vi "MB ICPCON Param redefine.vi"(6 "conninfo":T3={"host"="localhost", "port"="5432", "client_encoding"="WIN1251", "dbname"="data", "user"="postgres", "password"=""}, 7 "Status Reference":T1, 8 "error in (no error)":errorcluster, 9 "KFMTable":string="kfm_3", 10 "KFM param":string[](array[string]), 11 "KFM param in":T2) -> (0 "error":errorcluster, 3 "KFM param out":T2, 5 "Status Reference out":T1)   [LabVIEW 2019, in "ICPCON_Param.lvlib"]
uses:
  ICPCON_Param.lvlib
  ICPCON Param.ctl
  Eth timeouts.ctl
  Database/ctl/Coninfo.ctl
  Eth Status/Ctl/ICPCON Status.ctl
  MB_TCP2/MB_TCP_State.ctl
  KFMParamColumns.ctl
  Database/select_initial.vi
  <vilib>/Utility/error.llb/Clear Errors.vi
  Database/PostgreSQL2LabVIEW/libpqUtility64/src/PQgetTable.vi
  Database/PostgreSQL2LabVIEW/libpqUtility64/src/PQconnect.vi
  Database/PostgreSQL2LabVIEW/libpqUtility64/src/PQclose.vi
  Database/PostgreSQL2LabVIEW/libpqUtility64/src/PQfetchResultData.vi
  Database/PostgreSQL2LabVIEW/libpqlv64/src/PQresultErrorMessage.vi
  Database/PostgreSQL2LabVIEW/libpqlv64/src/PQresultStatus.vi
  Database/PostgreSQL2LabVIEW/libpqlv64/src/PQsendQuery.vi
  Database/PostgreSQL2LabVIEW/libpqlv64/src/PQgetResult.vi
  Database/PostgreSQL2LabVIEW/libpqUtility64/src/PQclear.vi
  Database/PostgreSQL2LabVIEW/libpqlv64/src/PQfinish.vi
  Database/PostgreSQL2LabVIEW/libpqlv64/src/PQconnectdb.vi
  Database/PostgreSQL2LabVIEW/libpqlv64/src/PQerrorMessage.vi
  Database/PostgreSQL2LabVIEW/libpqlv64/src/PQstatus.vi
  <vilib>/dlg_ctls.llb/Space Constant.vi
  Database/PostgreSQL2LabVIEW/libpqlv64/src/PQgetvalue.vi
  Database/PostgreSQL2LabVIEW/libpqlv64/src/PQnfields.vi
  Database/PostgreSQL2LabVIEW/libpqlv64/src/PQntuples.vi
  Database/PostgreSQL2LabVIEW/libpqlv64/src/PQclear.vi
  Eth Status/Eth Status.lvlib
  Database/PostgreSQL.lvlib
  MB_TCP2/MB_TCP.lvclass
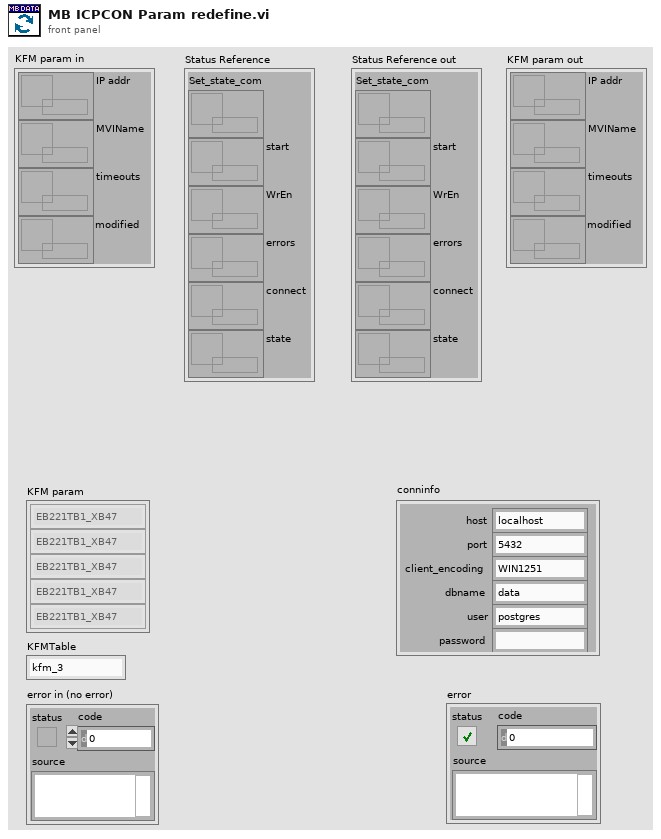
[diagram p1: front panel]
types:
  T1 = typedef "Eth Status.lvlib/ICPCON Status.ctl" = cluster{"Set_state_com":refnum<data-value>, "start":refnum<data-value>, "WrEn":refnum<data-value>, "errors":refnum<data-value>, "connect":refnum<data-value>, "state":refnum<data-value>}
  T2 = typedef "ICPCON_Param.lvlib/ICPCON Param.ctl" = cluster{"IP addr":refnum<data-value>, "MVIName":refnum<data-value>, "timeouts":refnum<data-value>, "modified":refnum<data-value>}
  T3 = typedef "PostgreSQL.lvlib/Coninfo.ctl" = cluster{"host":string, "port":string, "client_encoding":string, "dbname":string, "user":string, "password":string}
  T4 = typedef "ICPCON_Param.lvlib/KFMParamColumns.ctl" = enum16{"MVIName", "ip_adress", "port", "connection_timeout", "reconnection_timeout", "n_attempt_max", "reset_connect_timeout", "write_timeout", "read_timeout", "period", "enable", "write_enable"}
  T5 = typedef "ICPCON_Param.lvlib/Eth timeouts.ctl" = cluster{"conn_timeout":i32, "reconn_timeout":i32, "N attempt max":i32, "t_reset_TTL":i32, "write_timeout":i32, "read_timeout":i32, "period":i32}
  T6 = cluster{"Remote IP Address":string, "Remote Port":u16}[]
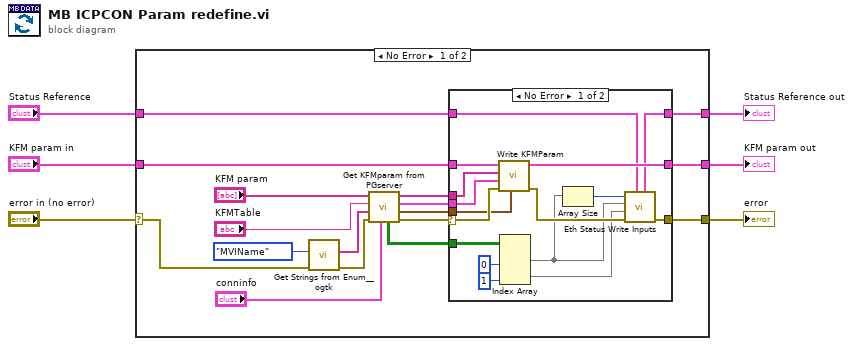
[diagram p0: block diagram]
diagram:
  n1 = case shown="No Error" "error in (no error)" {
    selector: "error in (no error)" -> [w8 w45]
    tunnel: [w23 w45] -> w6
    tunnel: "KFM param in" -> [w22 w44]
    tunnel: [w21 w44] -> w5
    tunnel: "Status Reference" -> [w20 w43]
    tunnel: [w19 w43] -> w1
    frame No Error {
      n2 = call <userlib>:"Get Strings from Enum__ogtk.vi"("error in (no error)"=w8, "Enum"=KFMParamColumns."MVIName" ("KFMParamColumns")) -> ("error out"=w7:errorcluster, "Enum Strings"=w9:string[])  [unwired: 6 in, 2 out]
      n3 = call "Get KFMparam from PGserver.vi"("conninfo"="conninfo", "error in (no error)"=w7, "KFMParamColumns"=w9, "KFMParamTable"="KFMTable", "KFMParameters"="KFM param") -> ("error out"=w15:errorcluster, "timeouts"=w12:T5[], "IP Address"=w16:T6, "MVIName"=w17:string[], "enable"=w11:bool[][])  [unwired: 2 in]
      n4 = case shown="No Error" w15 {
        selector: w15 -> [w38 w41]
        tunnel: w17 -> [w36 _]
        tunnel: w16 -> [w27 _]
        tunnel: [w33 w41] -> w23
        tunnel: w22 -> [w39 w42]
        tunnel: [w37 w42] -> w21
        tunnel: w12 -> [w35 _]
        tunnel: w11 -> [w29 _]
        tunnel: w20 -> [w32 w40]
        tunnel: [w24 w40] -> w19
        frame No Error {
          n5 = call "Write KFMParam.vi"("timeouts"=w35, "error in (no error)"=w38, "IP Address"=w27, "MVIName"=w36, "KFMParam in"=w39) -> ("error out"=w34:errorcluster, "KFMParam out"=w37:T2)  [unwired: 5 in]
          n6 = Index Array(array=w29, index (col) #1=0 ("index"), index (col) #2=1 ("index (col)")) -> (element #1=w25:bool[], element #2=w28:bool[])  [unwired: 2 in]
          n7 = Array Size(array=w25) -> (size(s)=w26:i32)
          n8 = call "Eth Status Write Inputs.vi"("Status Reference"=w32, "error in (no error)"=w34, "Write Enable"=w28, "Start"=w25, "Lenght"=w26) -> ("error out"=w33:errorcluster, "Status Reference out"=w24:T1)  [unwired: 5 in]
        }
        frame Error {
        }
      }
    }
    frame Error {
    }
  }
  "KFM param out" <- w5
  "error" <- w6
  "Status Reference out" <- w1
